vi "TCP Server Data Core.vi"(8 "error in (no error)":errorcluster, 9 "task (read)":T5, 10 "Data in":T1, 11 "Refnum":refnum<class "JKI TCP Server.lvclass">) -> (0 "error out":errorcluster, 2 "Data out":T1, 3 "dup Refnum":refnum<class "JKI TCP Server.lvclass">)   [LabVIEW 2020, in "JKI TCP Server.lvclass"]
doc: "LV2 Style Global for the GOOP data"
uses:
  JKI TCP Server.lvclass
  _Data Structures/TCP Server Data.ctl
  _Data Structures/TCP Server Listener Info Cluster.ctl
  _Data Structures/TCP Server Connection Info Cluster.ctl
  _Data Structures/TCP Server Handler RefNum.ctl
  _Data Structures/TCP Server Object Data Core Task Enum.ctl
  JKI TCP Server.lvclass/JKI TCP Server.ctl
panel:
  # "OpenGOOP Data Core.vi\n\nLV2 Style Global for the GOOP data\n\nCopyright (C) 2002 Jim Kring jim@jimkring.com\n\nPlease visit http://www.OpenG.org to learn about the\nOpen Source LabVIEW software movement.\n\nThis library is free software; you can redistribute it and/or\nmodify it under the terms of the GNU Lesser General Public\nLicense as published by the Free Software Foundation; either\nversion 2.1 of the License, or (at your option) any later version.\nThis library is distributed in the hope that it will be useful,\nbut WITHOUT ANY WARRANTY; without even the implied warranty of\nMERCHANTABILITY or FITNESS FOR A PARTICULAR PURPOSE. See the GNU\nLesser General Public License for more details.\nYou should have received a copy of the GNU Lesser General Public\nLicense along with this library; if not, write to the Free Software\nFoundation, Inc., 59 Temple Place, Suite 330, Boston, MA 02111-1307 USA"
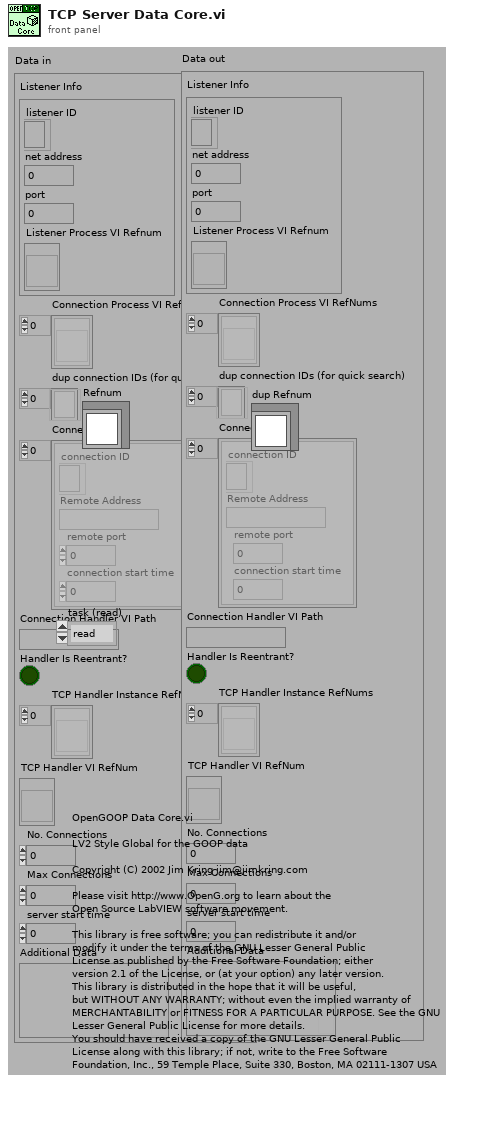
[diagram p1: front panel]
types:
  T1 = typedef "JKI TCP Server.lvclass/TCP Server Data.ctl" = cluster{"Listener Info":T2, "Connection Process VI RefNums":refnum<vi>[], "dup connection IDs (for quick search)":refnum<k5>[], "Connections":T3[], "Connection Handler VI Path":path, "Handler Is Reentrant?":bool, "TCP Handler Instance RefNums":T4[], "TCP Handler VI RefNum":T4, "No. Connections":u32, "Max Connections":u32, "server start time":u32, "Additional Data":variant}
  T2 = typedef "JKI TCP Server.lvclass/TCP Server Listener Info Cluster.ctl" = cluster{"listener ID":refnum<k5>, "net address":u32, "port":u16, "Listener Process VI Refnum":refnum<vi>}
  T3 = typedef "JKI TCP Server.lvclass/TCP Server Connection Info Cluster.ctl" = cluster{"connection ID":refnum<k5>, "Remote Address":string, "remote port":u16, "connection start time":u32}
  T4 = typedef "JKI TCP Server.lvclass/TCP Server Handler RefNum.ctl" = refnum<vi>
  T5 = typedef "JKI TCP Server.lvclass/TCP Server Object Data Core Task Enum.ctl" = enum16{"read", "write", "init"}
  T6 = typedef "JKI TCP Server.lvclass/TCP Server Object RefNum.ctl" = refnum<k1>
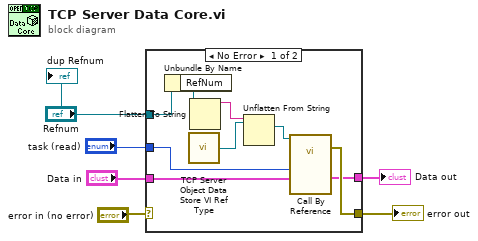
[diagram p0: block diagram]
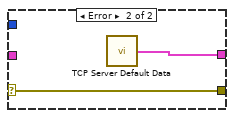
[diagram p2: hidden frame]
diagram:
  n1 = case shown="No Error" "error in (no error)" {
    selector: "error in (no error)" -> [_ w17]
    tunnel: "Refnum" -> [w8 _]
    tunnel: [w13 w17] -> w2
    tunnel: "Data in" -> [w10 _]
    tunnel: [w11 w16] -> w3
    tunnel: "task (read)" -> [w9 _]
    frame No Error {
      n2 = Unbundle By Name(w8) -> ("RefNum"=w7:T6)
      n3 = call "TCP Server Object Data Store VI Ref Type.vi"() -> ("VI Refnum (Object Data Store.vi Type)"=w12:refnum<vi>)  [unwired: 5 in]
      n4 = Flatten To String(anything=w7) -> (data string=w15:string)  [unwired: 3 in, 2 out]
      n5 = Unflatten From String(type=w12, binary string=w15) -> (value=w14:refnum<vi>)  [unwired: 3 in, 2 out]
      n6 = call-by-ref "?"(reference=w14, "Data in"=w10, "task (read)"=w9) -> (error out=w13:errorcluster, "Data in"=w11:T1)  [unwired: 10 in, 1 out]
    }
    frame Error {
      n7 = call "TCP Server Default Data.vi"() -> ("Data out"=w16:T1)
    }
  }
  "error out" <- w2
  "Data out" <- w3
  "dup Refnum" <- "Refnum"
